vi "Rate Limiter (DBL).vi"(2 "initialize":bool, 3 "dt":dbl format="%.6f", 4 "slew rate limit":T1 {"falling slew rate" format="%.2f"; "rising slew rate" format="%.2f"}, 5 "input point":dbl format="%.2f") -> (1 "output point":dbl format="%.2f")   [LabVIEW 2020, in "NI_AdvCtrl_nonlinear.lvlib"]
doc: "LabVIEW no longer supports this VI. You can obtain similar functionality by installing the LabVIEW Simulation Module.\n\nLimits the rate of change of a given signal."
uses:
  <vilib>/addons/control/advanced/NI_AdvCtrl_nonlinear.lvlib
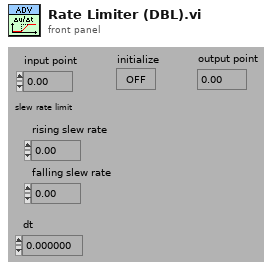
[diagram p1: front panel]
types:
  T1 = cluster{"rising slew rate":dbl, "falling slew rate":dbl}
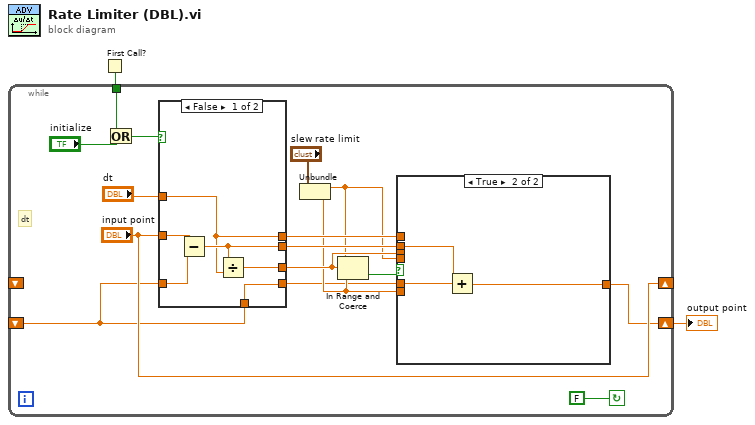
[diagram p0: block diagram]
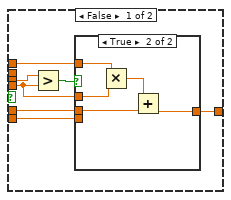
[diagram p2: hidden frame]
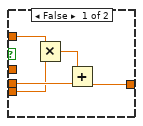
[diagram p3: hidden frame]
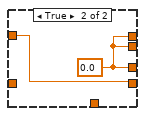
[diagram p4: hidden frame]
diagram:
  n1 = First Call?() -> (First Call?: T/F=w2:bool)
  n2 = while {
    shift-left: _ -> [w3]
    shift-right: [w5] -> w1
    tunnel: w2 -> [w13]
    shift-left: _ -> [_]
    shift-right: ["input point"] -> _
    stop <- FALSE continue-if-true
    # "dt"
    n3 = Or(x=w13, y="initialize") -> (x .or. y?=w11:bool)
    n4 = case shown="False" w11 {
      tunnel: [w39 w46] -> w4
      tunnel: w3 -> [w43 _]
      tunnel: "input point" -> [w44 w46]
      tunnel: "dt" -> [w40 _]
      tunnel: [w42 w45] -> w16
      tunnel: [w41 w45] -> w17
      tunnel: [w40 w45] -> w15
      tunnel: w3 -> [w39 _]
      frame False {
        n5 = Subtract(x=w44, y=w43) -> (x-y=w41:dbl)
        n6 = Divide(x=w41, y=w40) -> (x/y=w42:dbl)
      }
      frame True {
        w45 = 0.0
      }
    }
    n7 = Unbundle("slew rate limit") -> ("rising slew rate"=w8:dbl, "falling slew rate"=w7:dbl)
    n8 = In Range and Coerce(upper limit=w8, x=w16, lower limit=w7) -> (In Range?=w18:bool)  [unwired: 1 out]
    n9 = case shown="True" w18 {
      tunnel: w17 -> [_ w38]
      tunnel: w4 -> [w21 w37]
      tunnel: [w20 w36] -> w5
      tunnel: w16 -> [w25 _]
      tunnel: w8 -> [w22 _]
      tunnel: w15 -> [w23 _]
      tunnel: w7 -> [w19 _]
      frame False {
        n10 = Greater?(x=w25, y=w22) -> (0:w24:bool)
        n11 = case shown="True" w24 {
          tunnel: w23 -> [w30 w35]
          tunnel: w22 -> [_ w34]
          tunnel: w21 -> [w28 w32]
          tunnel: [w27 w31] -> w20
          tunnel: w19 -> [w26 _]
          frame False {
            n12 = Multiply(x=w30, y=w26) -> (x*y=w29:dbl)
            n13 = Add(x=w29, y=w28) -> (x+y=w27:dbl)
          }
          frame True {
            n14 = Multiply(x=w35, y=w34) -> (x*y=w33:dbl)
            n15 = Add(x=w33, y=w32) -> (x+y=w31:dbl)
          }
        }
      }
      frame True {
        n16 = Add(x=w38, y=w37) -> (x+y=w36:dbl)
      }
    }
  }
  "output point" <- w1
